vi "Add Channel.vi"(4 "Property Values":variant[](array[variant]), 6 "Property names":string[](array[string]), 7 "Highlight? (F)":bool, 8 "error in":errorcluster, 9 "Channel":T1, 10 "Name":string, 11 "Frame Ref":T3 format="%.0x") -> (0 "error out":errorcluster, 3 "Channel Ref out":T3 format="%.0x")   [LabVIEW 2020, in "Communication Bus Template Scripting.lvlib"]
uses:
  Communication Bus Template Scripting.lvlib
  <vilib>/NI VeriStand/Custom Device API/Custom Device API.lvlib
  Constants.vi
  <vilib>/NI VeriStand/Custom Device API/Custom Device Item Ref.ctl
  <vilib>/NI VeriStand/Custom Device API/Custom Device Channel Type.ctl
  <vilib>/NI VeriStand/Custom Device API/Custom Device Channel.ctl
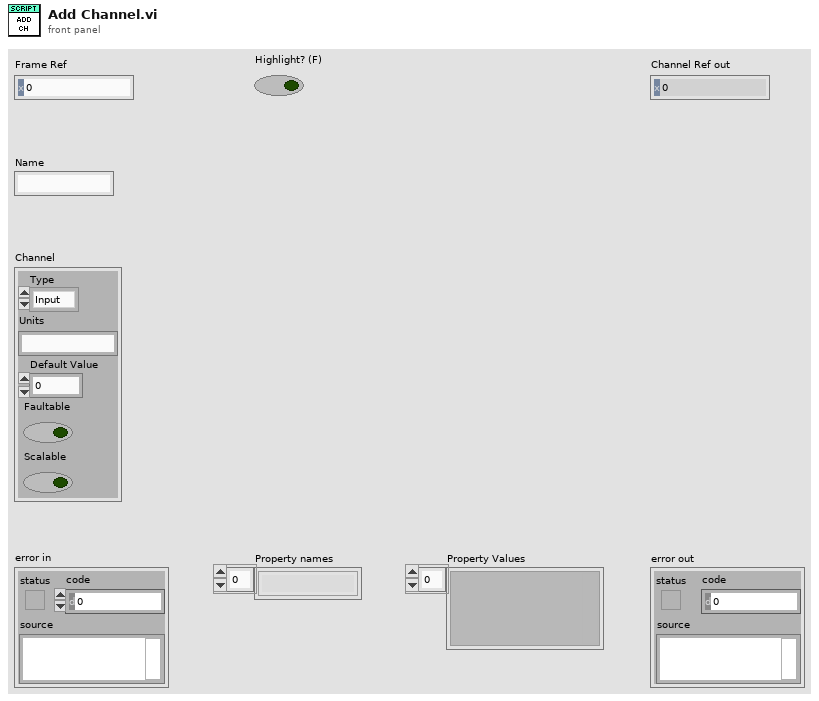
[diagram p1: front panel]
types:
  T1 = typedef "Custom Device API.lvlib/Custom Device Channel.ctl" = cluster{"Type":T2, "Units":string, "Default Value":dbl, "Faultable":bool, "Scalable":bool}
  T2 = typedef "Custom Device API.lvlib/Custom Device Channel Type.ctl" = enum16{"Input", "Output"}
  T3 = typedef "Custom Device API.lvlib/Custom Device Item Ref.ctl" = u64
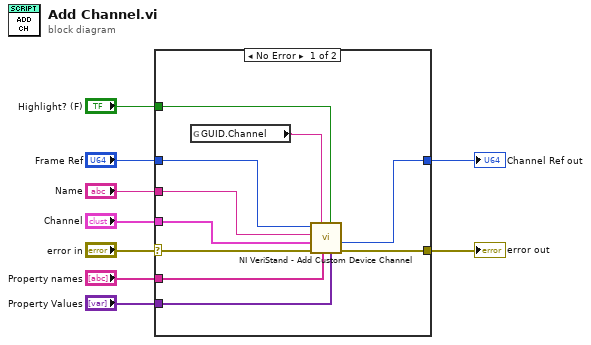
[diagram p0: block diagram]
diagram:
  n1 = case shown="No Error" "error in" {
    selector: "error in" -> [w19 w20]
    tunnel: [w18 w20] -> w8
    tunnel: "Frame Ref" -> [w16 _]
    tunnel: [w15 _] -> w6
    tunnel: "Name" -> [w17 _]
    tunnel: "Channel" -> [w14 _]
    tunnel: "Highlight? (F)" -> [w13 _]
    tunnel: "Property Values" -> [w11 _]
    tunnel: "Property names" -> [w10 _]
    frame No Error {
      n2 = global read "Constants.vi" "GUID.Channel"() -> (w12:string)
      n3 = call <vilib>:"NI VeriStand - Add Custom Device Channel.vi"("Property Values"=w11, "Highlight? (F)"=w13, "Property names"=w10, "GUID (Default Channel)"=w12, "error in (no error)"=w19, "Channel"=w14, "Channel Name"=w17, "Parent Ref in"=w16) -> ("error out"=w18:errorcluster, "Channel Ref"=w15:T3)  [unwired: 2 out]
    }
    frame Error {
    }
  }
  "Channel Ref out" <- w6
  "error out" <- w8
